vi "Create datalog header string.vi"() -> (0 "Datalog header string":string)   [LabVIEW 2017]
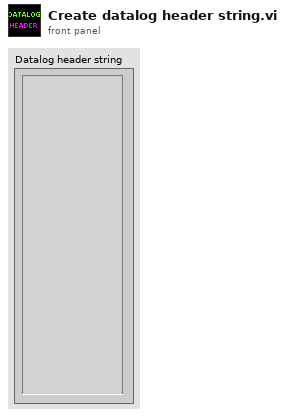
[diagram p1: front panel]
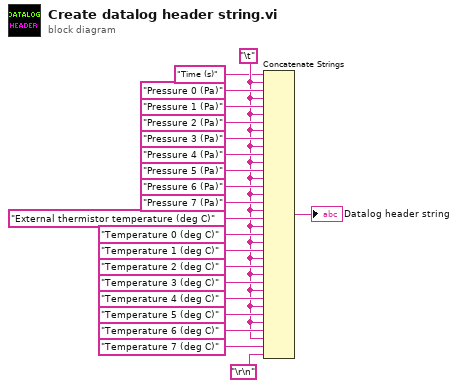
[diagram p0: block diagram]
diagram:
  w2 = "\t"
  n1 = Concatenate Strings("Time (s)", w2, "Pressure 0 (Pa)", w2, "Pressure 1 (Pa)", w2, "Pressure 2 (Pa)", w2, "Pressure 3 (Pa)", w2, "Pressure 4 (Pa)", w2, "Pressure 5 (Pa)", w2, "Pressure 6 (Pa)", w2, "Pressure 7 (Pa)", w2, "External thermistor temperature (deg C)", w2, "Temperature 0 (deg C)", w2, "Temperature 1 (deg C)", w2, "Temperature 2 (deg C)", w2, "Temperature 3 (deg C)", w2, "Temperature 4 (deg C)", w2, "Temperature 5 (deg C)", w2, "Temperature 6 (deg C)", w2, "Temperature 7 (deg C)", "\r\n") -> (→"Datalog header string":string)
